vi "ith HTL.vi"(0 "HTL Array":dbl[][](array[numeric]), 2 "File Info input":T1={"FilePath"=path "/DATA/Labview Items", "Field (T)"=55.0, "Temperature (K)"=77.0, "X-Axis"=enum."nm", "Center nm"=55.0, "Current Grating Density"=enum."600", "CCD Parameters"={"Exposure Time (s)"=0.2, "Offset"=0.0, "BkgrdCrct"=FALSE, "Shutter"=FALSE, "Mode"=enum."Regular", "Repetition"=4, "dt or s"=0.0}, "Operation Mode"=enum."NML Data Acquisition", "Exp Index"=0, "Index_repetition"=0, "Index"=0, "Current Detector"=enum."CCD-1024x256"} {"CCD Parameters"."dt or s" format="%#.6f"; "CCD Parameters"."Repetition" min=1; "CCD Parameters"."Offset" format="%#.2f"; "CCD Parameters"."Exposure Time (s)" min=0.02 max=6000.0 format="%#.2f"; "Center nm" format="%.2f"; "Temperature (K)" format="%.2f"; "Field (T)" format="%.2f"}, 3 "Prefix Indexed":bool=TRUE caption="Prefix indexed", 5 "SubFolderNamesArray":string[](array[string]), 11 "error in":errorcluster, 12 "Path array":path[](array[path]), 14 "File Path Parameter":T7={"Filename Prefix"="MyData", "Extension"=enum."±Field", "Suffix"="", "Current Path"=path "/opticsdata/Users"}) -> (4 "Stop?":bool, 8 "File Info output":T1={"FilePath"=path "/DATA/Labview Items", "Field (T)"=55.0, "Temperature (K)"=77.0, "X-Axis"=enum."nm", "Center nm"=55.0, "Current Grating Density"=enum."600", "CCD Parameters"={"Exposure Time (s)"=0.2, "Offset"=0.0, "BkgrdCrct"=FALSE, "Shutter"=FALSE, "Mode"=enum."Regular", "Repetition"=4, "dt or s"=0.0}, "Operation Mode"=enum."NML Data Acquisition", "Exp Index"=0, "Index_repetition"=0, "Index"=0, "Current Detector"=enum."CCD-1024x256"} {"CCD Parameters"."dt or s" format="%#.6f"; "CCD Parameters"."Repetition" min=1; "CCD Parameters"."Offset" format="%#.2f"; "CCD Parameters"."Exposure Time (s)" min=0.02 max=6000.0 format="%#.2f"; "Center nm" format="%.2f"; "Temperature (K)" format="%.2f"; "Field (T)" format="%.2f"}, 15 "error out":errorcluster)   [LabVIEW 2019]
doc: "This Vi extract current field and set the scan continue boolean variable.\n\nThe field step can be either positive or negative.\n\nIf any of the absolute field value exceeds the maximum allowed limit, it will be replaced with the maximum field value itself"
uses:
  Globals and TypeDefs/Type Definitions.llb/FilePathParameter.ctt
  Globals and TypeDefs/Type Definitions.llb/FileInfoParameter.ctt
  Globals and TypeDefs/Type Definitions.llb/Wavelength Unit.ctt
  Globals and TypeDefs/Type Definitions.llb/McPherson Grating Density.ctl
  Globals and TypeDefs/Type Definitions.llb/CCDParameter.ctt
  Globals and TypeDefs/Type Definitions.llb/OperationMode.ctt
  Globals and TypeDefs/Type Definitions.llb/ListOfDetectors.ctt
  Globals and TypeDefs/gTemperature.vi
  Globals and TypeDefs/gSpectrometer.vi
  Globals and TypeDefs/gHField.vi
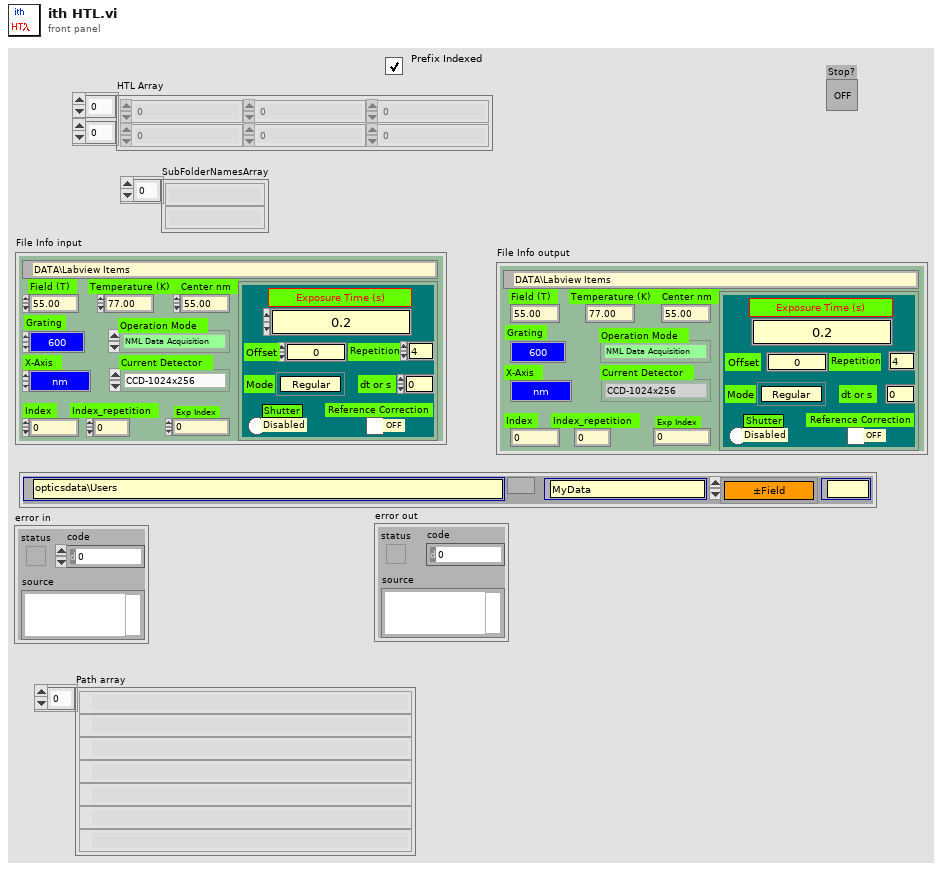
[diagram p1: front panel]
types:
  T1 = typedef "FileInfoParameter.ctt" = cluster{"FilePath":path, "Field (T)":dbl, "Temperature (K)":dbl, "X-Axis":T2, "Center nm":dbl, "Current Grating Density":T3, "CCD Parameters":T4, "Operation Mode":T5, "Exp Index":u32, "Index_repetition":u16, "Index":u16, "Current Detector":T6}
  T2 = typedef "Wavelength Unit.ctt" = enum8{"Point", "nm", "eV", "meV", "cm_1"}
  T3 = typedef "McPherson Grating Density.ctl" = enum8{"150", "300", "600", "1200", "1800"}
  T4 = typedef "CCDParameter.ctt" = cluster{"Exposure Time (s)":dbl, "Offset":dbl, "BkgrdCrct":bool, "Shutter":bool, "Mode":enum8{"Regular", "OverExp Cor", "SpikeRemove", "ForCalibration"}, "Repetition":u16, "dt or s":dbl}
  T5 = typedef "OperationMode.ctt" = enum16{"Standby", "CCD Single Shot", "CCD Sequence Shots", "CCD Custom Shots", "CCD Reference Shot", "Step Scanning ", "Time Scanning", "NML Data Acquisition"}
  T6 = typedef "ListOfDetectors.ctt" = enum8{"CCD-1024x256", "InGaAs PDA-1024x1", "CCD-1340x400", "Ge Single Channel", "Si Single Channel", "PMT Single Channel"}
  T7 = typedef "FilePathParameter.ctt" = cluster{"Filename Prefix":string, "Extension":enum16{"none", "\".001\",\".002\", ...", "001 (No dot)", "±Field", "pField nField", "Temperature", "Wavelength", "T(K)±H(T)", "(nm)T(K)±H(T)", "User Defined"}, "Suffix":string, "Current Path":path}
  T8 = enum8{"Regular", "OverExp Cor", "SpikeRemove", "ForCalibration"}
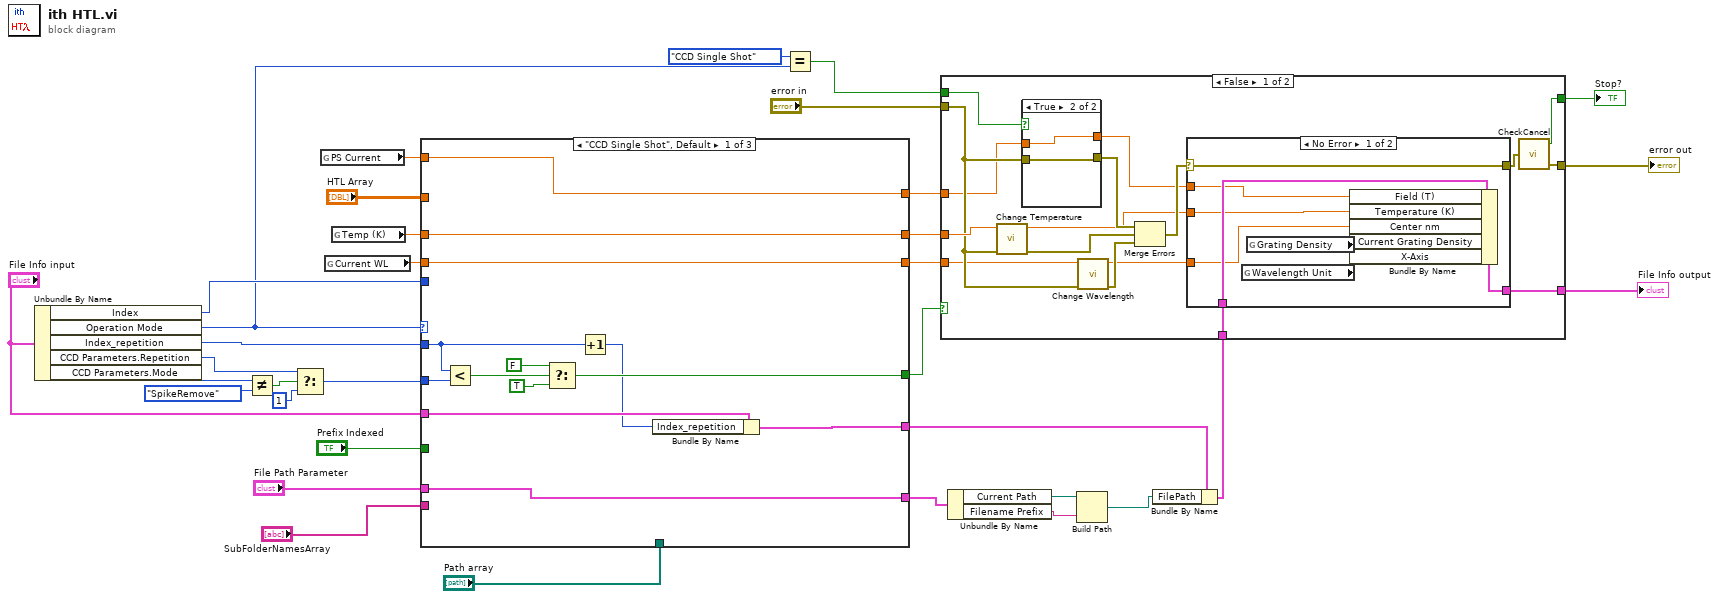
[diagram p0: block diagram]
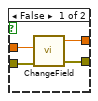
[diagram p2: hidden frame]
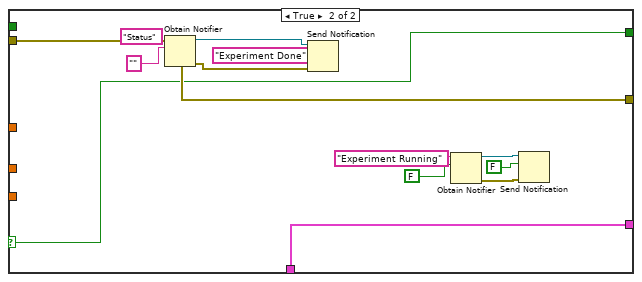
[diagram p4: hidden frame]
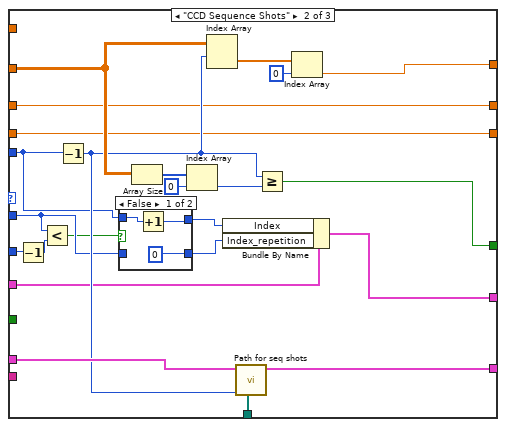
[diagram p5: hidden frame]
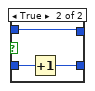
[diagram p6: hidden frame]
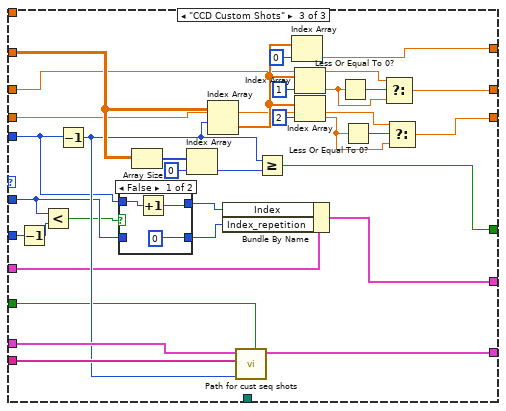
[diagram p7: hidden frame]
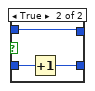
[diagram p8: hidden frame]
diagram:
  n1 = Unbundle By Name("File Info input") -> ("Index"=w17:u16, "Operation Mode"=w3:T5, "Index_repetition"=w10:u16, "CCD Parameters.Repetition"=w23:u16, "CCD Parameters.Mode"=w20:T8)
  n2 = Not Equal?(x=w20, y=T8."SpikeRemove") -> (x != y?=w22:bool)
  n3 = Select(t=w23, s=w22, f=u8 1) -> (s? t:f=w9:u16)
  n4 = global read "gHField.vi" "PS Current"() -> (w11:dbl)
  n5 = global read "gSpectrometer.vi" "Current WL"() -> (w12:dbl)
  n6 = global read "gTemperature.vi" "Temp (K)"() -> (w13:dbl)
  n7 = case shown="\"CCD Single Shot\", Default" w3 {
    tunnel: "File Info input" -> [w43 w58 w93]
    tunnel: "HTL Array" -> [_ w65 w101]
    tunnel: w17 -> [_ w59 w94]
    tunnel: [w47 w60 w95] -> w33
    tunnel: [w38 w64 w100] -> w29
    tunnel: [w40 w54 w84] -> w28
    tunnel: [w39 w53 w79] -> w27
    tunnel: "SubFolderNamesArray" -> [_ _ w99]
    tunnel: "File Path Parameter" -> [w46 w63 w98]
    tunnel: [w46 w62 w97] -> w19
    tunnel: w10 -> [w35 w50 w86]
    tunnel: [w41 w55 w90] -> w15
    tunnel: "Prefix Indexed" -> [_ _ w89]
    tunnel: w13 -> [w40 w54 w81]
    tunnel: w12 -> [w39 w53 w77]
    tunnel: w11 -> [w38 _ _]
    tunnel: w9 -> [w37 w52 w87]
    tunnel: "Path array" -> [_ w48 _]
    frame "CCD Single Shot", Default {
      n8 = Less?(x=w35, y=w37) -> (x < y?=w36:bool)
      n9 = Select(t=FALSE, s=w36, f=TRUE ("Stop?")) -> (s? t:f=w47:bool)
      n10 = Increment(x=w35) -> (x+1=w42:u16)
      n11 = Bundle By Name(cluster=w43, "Index_repetition"=w42) -> (w41:T1)
    }
    frame "CCD Sequence Shots" {
      n12 = Decrement(x=w52) -> (x-1=w51:u16)
      n13 = Less?(x=w50, y=w51) -> (x < y?=w49:bool)
      n14 = Decrement(x=w59) -> (x-1=w61:u16)
      n15 = case shown="False" w49 {
        tunnel: w59 -> [w73 w75]
        tunnel: w50 -> [_ w76]
        tunnel: [w72 w75] -> w57
        tunnel: [u16 0 ("Index_repetition") w74] -> w56
        frame False {
          n16 = Increment(x=w73) -> (x+1=w72:u16)
        }
        frame True {
          n17 = Increment(x=w76) -> (x+1=w74:u16)
        }
      }
      n18 = Array Size(array=w65) -> (size(s)=w66:i32[])
      n19 = Index Array(array=w66, index=0) -> (element=w68:i32)
      n20 = Index Array(array=w65, index (row)=w61) -> (element=w69:dbl[])  [unwired: 1 in]
      n21 = Bundle By Name(cluster=w58, "Index"=w57, "Index_repetition"=w56) -> (w55:T1)
      n22 = call "Path for seq shots.vi"("Path array"=w48, "Index"=w61, "File Path Input"=w63) -> ("File Path output"=w62:T7)  [unwired: 6 in]
      n23 = Greater Or Equal?(x=w61, y=w68) -> (x >= y?=w60:bool)
      n24 = Index Array(array=w69, index=0) -> (element=w64:dbl)
    }
    frame "CCD Custom Shots" {
      n25 = Decrement(x=w87) -> (x-1=w88:u16)
      n26 = Less?(x=w86, y=w88) -> (x < y?=w85:bool)
      n27 = Decrement(x=w94) -> (x-1=w96:u16)
      n28 = case shown="False" w85 {
        tunnel: w94 -> [w111 w113]
        tunnel: w86 -> [_ w114]
        tunnel: [w110 w113] -> w92
        tunnel: [u16 0 ("Index_repetition") w112] -> w91
        frame False {
          n29 = Increment(x=w111) -> (x+1=w110:u16)
        }
        frame True {
          n30 = Increment(x=w114) -> (x+1=w112:u16)
        }
      }
      n31 = Array Size(array=w101) -> (size(s)=w102:i32[])
      n32 = Index Array(array=w102, index=0) -> (element=w104:i32)
      n33 = Index Array(array=w101, index (row)=w96) -> (element=w105:dbl[])  [unwired: 1 in]
      n34 = Bundle By Name(cluster=w93, "Index"=w92, "Index_repetition"=w91) -> (w90:T1)
      n35 = call "Path for cust seq shots.vi"("Diff Prefix?"=w89, "Index"=w96, "SubfolderName"=w99, "File Path Input"=w98) -> ("File Path output"=w97:T7)  [unwired: 5 in]
      n36 = Greater Or Equal?(x=w96, y=w104) -> (x >= y?=w95:bool)
      n37 = Index Array(array=w105, index=0) -> (element=w100:dbl)
      n38 = Index Array(array=w105, index=1) -> (element=w82:dbl)
      n39 = Index Array(array=w105, index=2) -> (element=w78:dbl)
      n40 = Less Or Equal To 0?(x=w82) -> (x <= 0?=w83:bool)
      n41 = Less Or Equal To 0?(x=w78) -> (x <= 0?=w80:bool)
      n42 = Select(t=w81, s=w83, f=w82) -> (s? t:f=w84:dbl)
      n43 = Select(t=w77, s=w80, f=w78) -> (s? t:f=w79:dbl)
    }
  }
  n44 = Equal?(x=OperationMode.ctt."CCD Single Shot", y=w3) -> (x = y?=w1:bool)
  n45 = Unbundle By Name(w19) -> ("Current Path"=w7:path, "Filename Prefix"=w6:string)
  n46 = Build Path(base path=w7, name or relative path=w6) -> (appended path=w5:path)
  n47 = Bundle By Name(cluster=w15, "FilePath"=w5) -> (w18:T1)
  n48 = case shown="False" w33 {
    selector: w33 -> [_ w148]
    tunnel: w28 -> [w131 _]
    tunnel: [w117 w160] -> w31
    tunnel: "error in" -> [w127 w160]
    tunnel: w18 -> [w129 w159]
    tunnel: [w128 w159] -> w30
    tunnel: w29 -> [w126 _]
    tunnel: w27 -> [w125 _]
    tunnel: [w116 w148] -> w4
    tunnel: w1 -> [w115 _]
    frame False {
      n49 = call "Change Temperature.vi"("error in"=w127, "GOTO"=w131) -> ("error out"=w123:errorcluster, "Final Temperature"=w120:dbl)  [unwired: 7 in]
      n50 = case shown="True" w115 {
        tunnel: w127 -> [w135 w137]
        tunnel: w126 -> [w134 w136]
        tunnel: [w133 w137] -> w124
        tunnel: [w132 w136] -> w121
        frame False {
          n51 = call "ChangeField.vi"("Desired Field (T)"=w134, "error in (no error)"=w135) -> ("Tesla"=w132:dbl, "error out"=w133:errorcluster)  [unwired: 4 in, 1 out]
        }
        frame True {
        }
      }
      n52 = call "Change Wavelength.vi"("error in"=w127, "GOTO"=w125) -> ("error out"=w122:errorcluster, "Final nm"=w119:dbl)  [unwired: 6 in, 1 out]
      n53 = Merge Errors(w124, w123, w122) -> (w130:errorcluster)
      n54 = case shown="No Error" w130 {
        selector: w130 -> [w145 w147]
        tunnel: [w145 w147] -> w118
        tunnel: w129 -> [w144 w146]
        tunnel: [w140 w146] -> w128
        tunnel: w121 -> [w143 _]
        tunnel: w120 -> [w142 _]
        tunnel: w119 -> [w141 _]
        frame No Error {
          n55 = global read "gSpectrometer.vi" "Wavelength Unit"() -> (w138:T2)
          n56 = global read "gSpectrometer.vi" "Grating Density"() -> (w139:T3)
          n57 = Bundle By Name(cluster=w144, "Field (T)"=w143, "Temperature (K)"=w142, "Center nm"=w141, "Current Grating Density"=w139, "X-Axis"=w138) -> (w140:T1)
        }
        frame Error {
        }
      }
      n58 = call "CheckCancel.vi"("error in (no error)"=w118) -> ("Cancelled"=w116:bool, "error out"=w117:errorcluster)  [unwired: 1 in]
    }
    frame True {
      n59 = Obtain Notifier(name (unnamed)="Status", notification data type="" ("Status")) -> (notifier out=w150:refnum<notifier>, error out=w149:errorcluster)  [unwired: 2 in, 1 out]
      n60 = Send Notification(notification="Experiment Done", notifier=w150, error in (no error)=w149) -> ()  [unwired: 2 out]
      n61 = Obtain Notifier(name (unnamed)="Experiment Running", notification data type=FALSE ("SaveData?")) -> (notifier out=w156:refnum<notifier>, error out=w157:errorcluster)  [unwired: 2 in, 1 out]
      n62 = Send Notification(notification=FALSE, notifier=w156, error in (no error)=w157) -> ()  [unwired: 2 out]
    }
  }
  "File Info output" <- w30
  "Stop?" <- w4
  "error out" <- w31
